vi "C884Config.vi"(0 "All axes? Refnum":refnum<vi>, 1 "Stages Selection Refnum":refnum<vi>, 2 "Position Refnum":refnum<vi>, 3 "Identification Refnum":refnum<vi>, 4 "Referencing successful Refnum":refnum<vi>, 5 "Host Addresss Refnum":refnum<vi>, 6 "Message Out Refnum":refnum<vi>, 7 "+/- mvt range Refnum":refnum<vi>, 8 "Axes to Move Refnum":refnum<vi>, 9 "Connected Axes Refnum":refnum<vi>, 10 "Referencing mode":T1(array[ring])=[enum."FRF (-> FNL)", enum."FRF (-> FNL)", enum."FRF (-> FNL)", enum."FRF (-> FNL)"], 11 "Error OUT Refnum":refnum<vi>, 12 "En cours LED Refnum":refnum<vi>, 13 "LED Initialis. OK? Refnum":refnum<vi>) -> ()   [LabVIEW 2014]
panel:
  out "+/- movement\nrange":dbl[](array[numeric]) format="%.6f"
  out "error out":errorcluster
  out "Identification":string
  out "Referencing\nsuccessful?":bool[](array[boolean])
  out "Conn. \nAxes":string[](array[string])
  out "Position":dbl[](array[numeric]) format="%.6f"
  out "TCP/IP settings.Host address/name":string
  # "If yes:"
  # "If not:"
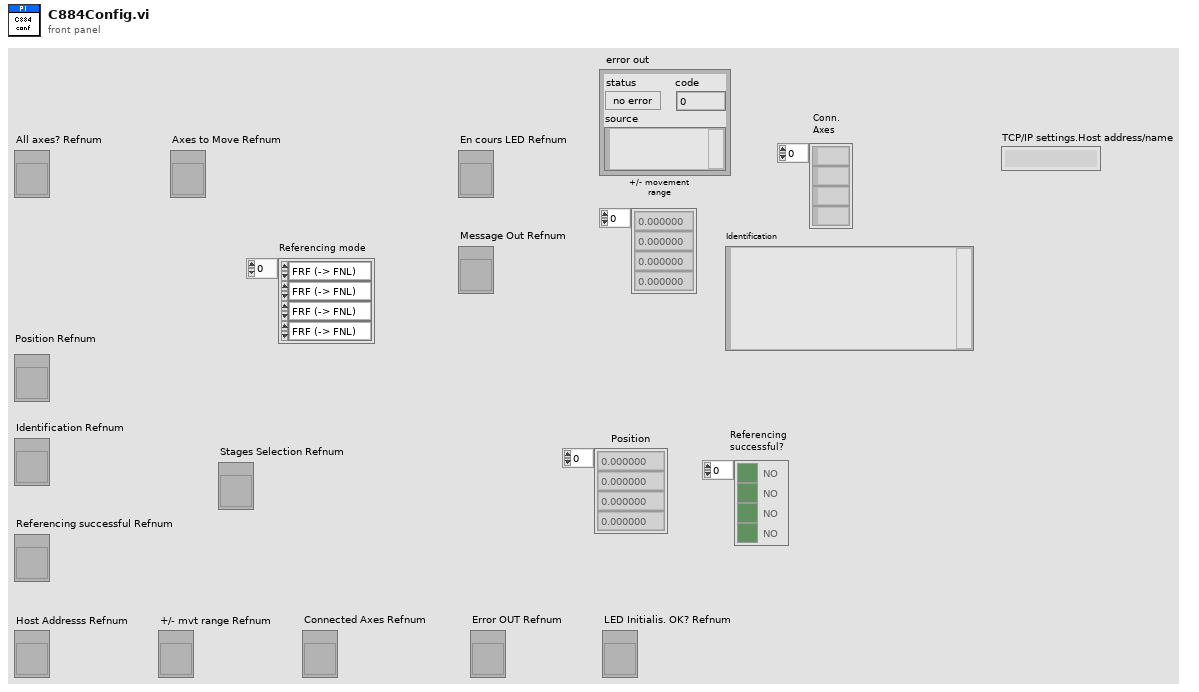
[diagram p1: front panel]
types:
  T1 = enum16{"FRF (-> FNL)", "FRF", "FNL", "FPL", "RON OFF"}[]
  T2 = cluster{"Check FRF?":bool, "Referencing mode":enum16{"FRF (-> FNL)", "FRF", "FNL", "FPL", "RON OFF"}[]}
  T3 = cluster{"RS232 settings":cluster{"Portnumber":i32, "Baudrate":u16}, "TCP/IP settings":cluster{"Host address/name":string, "Port":i32, "Board":i32, "TCP/IP Search?":bool}, "USB settings":cluster{"S/N":string, "USB Search?":bool}}
  T4 = cluster{"Force?":bool, "Dialog?":bool, "Stages":string[]}
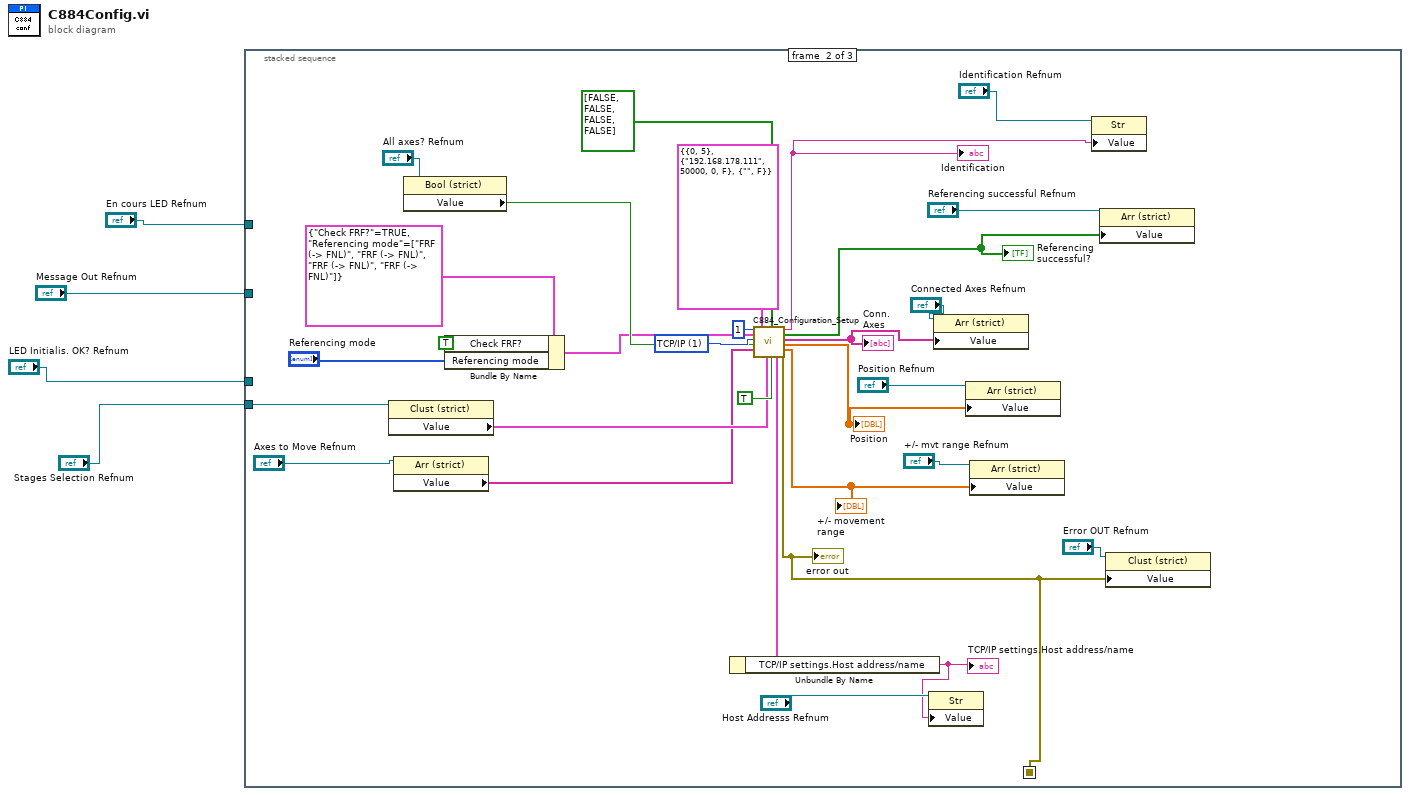
[diagram p0: block diagram]
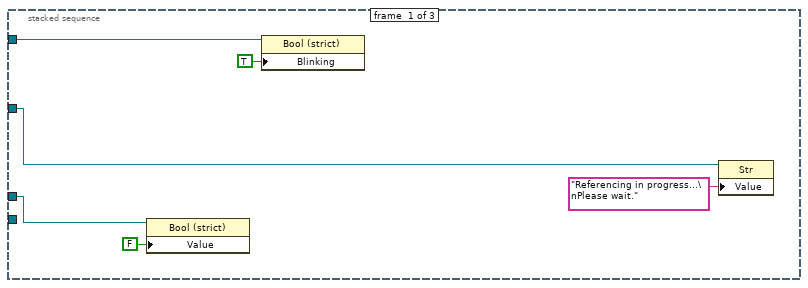
[diagram p2: hidden frame]
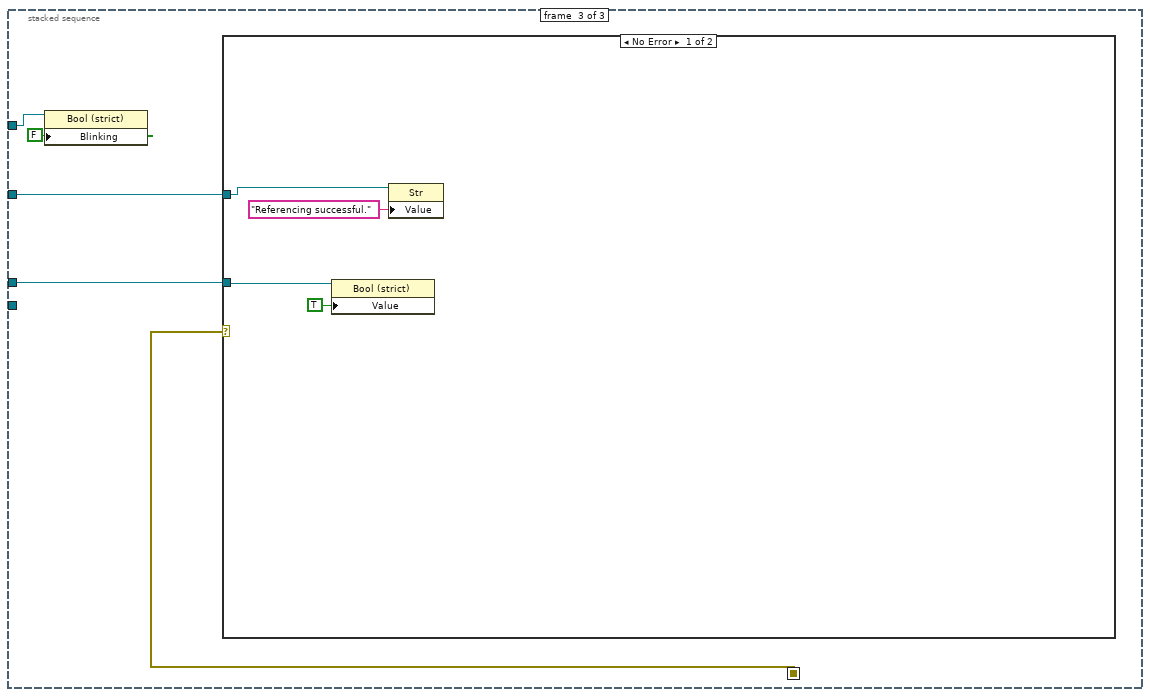
[diagram p3: hidden frame]
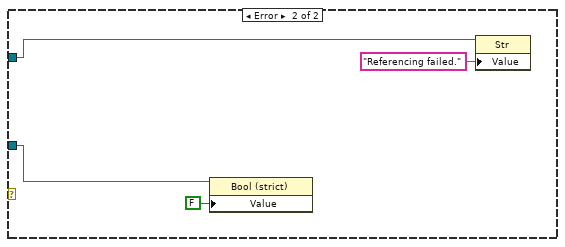
[diagram p4: hidden frame]
diagram:
  n1 = stacked-sequence {
    seq-local: [_ w20 _] -> [_ _ w43]
    tunnel: "En cours LED Refnum" -> [w9 _ w44]
    tunnel: "Message Out Refnum" -> [w8 _ w42]
    tunnel: "LED Initialis. OK? Refnum" -> [w6 _ w41]
    tunnel: "Stages Selection Refnum" -> [_ w17 _]
    frame #0 {
      n2 = property class="Bool (strict)"(reference=w6, "Value"=FALSE) -> ()  [unwired: 1 in, 2 out]
      n3 = property class="Bool (strict)"(reference=w9, "Blinking"=TRUE) -> ()  [unwired: 1 in, 2 out]
      n4 = property class="Str"(reference=w8, "Value"="Referencing in progress...\nPlease wait.") -> ()  [unwired: 1 in, 2 out]
    }
    frame #1 {
      w37 = u16 1 items=["RS232", "TCP/IP", "USB"] ("Interface")
      n5 = property class="Clust (strict)"(reference=w17) -> ("Value"=w16:T4)  [unwired: 1 in, 2 out]
      n6 = property class="Arr (strict)"(reference="Axes to Move Refnum") -> ("Value"=w15:string[])  [unwired: 1 in, 2 out]
      n7 = property class="Bool (strict)"(reference="All axes? Refnum") -> ("Value"=w34:bool)  [unwired: 1 in, 2 out]
      n8 = Bundle By Name(cluster=T2 {"Check FRF?"=TRUE, "Referencing mode"=[enum."FRF (-> FNL)", enum."FRF (-> FNL)", enum."FRF (-> FNL)", enum."FRF (-> FNL)"]} ("Referencing"), "Check FRF?"=TRUE, "Referencing mode"="Referencing mode") -> (w11:T2)
      n9 = call "C884_Configuration_Setup.vi"("System no."=1, "Referencing"=w11, "Interface"=w37, "All axes?"=w34, "Axes to move"=w15, "Interface settings"=T3 {"RS232 settings"={"Portnumber"=0, "Baudrate"=5}, "TCP/IP settings"={"Host address/name"="192.168.178.111", "Port"=50000, "Board"=0, "TCP/IP Search?"=FALSE}, "USB settings"={"S/N"="", "USB Search?"=FALSE}}, "Stage selection"=w16, "Move to middle?"=bool[] [FALSE, FALSE, FALSE, FALSE], "Switch servo on?"=TRUE) -> ("Interface settings out"=w38:T3, "Identification"=w21:string, "Referencing\nsuccessful?"=w23:bool[], "Conn. \nAxes"=w25:string[], "Position"=w27:dbl[], "+/- movement\nrange"=w29:dbl[], "error out"=w20:errorcluster)  [unwired: 4 in]
      "Position" <- w27
      "Conn. \nAxes" <- w25
      "Referencing\nsuccessful?" <- w23
      "Identification" <- w21
      "error out" <- w20
      "+/- movement\nrange" <- w29
      n10 = Unbundle By Name(w38) -> ("TCP/IP settings.Host address/name"=w32:string)
      "TCP/IP settings.Host address/name" <- w32
      n11 = property class="Str"(reference="Host Addresss Refnum", "Value"=w32) -> ()  [unwired: 1 in, 2 out]
      n12 = property class="Arr (strict)"(reference="Connected Axes Refnum", "Value"=w25) -> ()  [unwired: 1 in, 2 out]
      n13 = property class="Arr (strict)"(reference="Position Refnum", "Value"=w27) -> ()  [unwired: 1 in, 2 out]
      n14 = property class="Arr (strict)"(reference="+/- mvt range Refnum", "Value"=w29) -> ()  [unwired: 1 in, 2 out]
      n15 = property class="Str"(reference="Identification Refnum", "Value"=w21) -> ()  [unwired: 1 in, 2 out]
      n16 = property class="Arr (strict)"(reference="Referencing successful Refnum", "Value"=w23) -> ()  [unwired: 1 in, 2 out]
      n17 = property class="Clust (strict)"(reference="Error OUT Refnum", "Value"=w20) -> ()  [unwired: 1 in, 2 out]
    }
    frame #2 {
      n18 = property class="Bool (strict)"(reference=w44, "Blinking"=FALSE) -> ()  [unwired: 1 in, 2 out]
      n19 = case shown="No Error" w43 {
        tunnel: w42 -> [w49 w52]
        tunnel: w41 -> [w46 w50]
        frame No Error {
          n20 = property class="Bool (strict)"(reference=w46, "Value"=TRUE) -> ()  [unwired: 1 in, 2 out]
          n21 = property class="Str"(reference=w49, "Value"="Referencing successful.") -> ()  [unwired: 1 in, 2 out]
        }
        frame Error {
          n22 = property class="Bool (strict)"(reference=w50, "Value"=FALSE) -> ()  [unwired: 1 in, 2 out]
          n23 = property class="Str"(reference=w52, "Value"="Referencing failed.") -> ()  [unwired: 1 in, 2 out]
        }
      }
    }
  }
